vi "S&E Monitor.vi"(1 "Action(GET 250)":T3=enum."Get last  250", 5 "Type":T1, 7 "E&S Message in":T2, 11 "error in (no error)":errorcluster, 12 "Numb Alarm(250)":i32=250) -> (8 "S&E":T2[](array[typedef]), 15 "error out":errorcluster)   [LabVIEW 2011]
uses:
  Actino S&E monitor.ctl
  emi Lib/System 01/0 - General/S&E reporting/Private/_emi_ S&E Message.ctl
  emi Lib/System 01/0 - General/S&E reporting/Private/_emi_ S&E Message type.ctl
  reate/S&E Analog Alarm type.ctl
  GUI/Status Indikator Helper.ctl
  reate/S&E Digital Alarm Type.ctl
  Measurments Handling/Status Digitalish.ctl
  <vilib>/Utility/VariantDataType/GetNumericInfo.vi
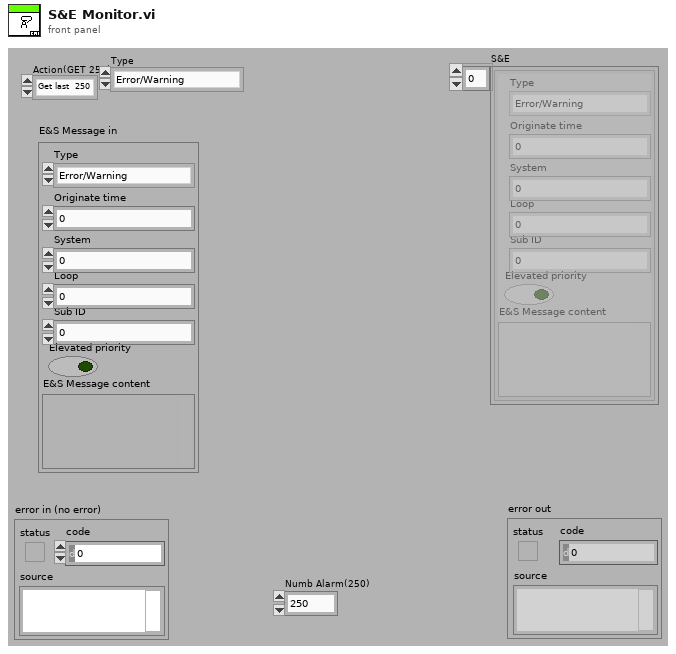
[diagram p1: front panel]
types:
  T1 = typedef "_emi_ S&E Message type.ctl" = enum16{"Error/Warning", "Note", "Debug", "Event", "Alarm Analog", "Alarm Digital", "Annotation"}
  T2 = typedef "_emi_ S&E Message.ctl" = cluster{"Type":T1, "Originate time":dbl, "System":u8, "Loop":u16, "Sub ID":u16, "Elevated priority":bool, "E&S Message content":variant}
  T3 = typedef "Actino S&E monitor.ctl" = enum16{"GET(type history)", "SET S&E", "(Re)Init", "Get Error state", "Get  Alarm state", "Get All", "Get last  250", "Get Alarm History"}
  T4 = typedef "S&E Analog Alarm type.ctl" = cluster{"Alarm":bool, "State":T5, "Value":dbl, "Source name":string}
  T5 = typedef "Status Indikator Helper.ctl" = enum16{"Norm", "L", "H", "LL", "HH", "Value", "Technical"}
  T6 = typedef "S&E Digital Alarm Type.ctl" = cluster{"Alarm":bool, "Enum":T5, "Value":T7, "Source name":string, "Status text":string}
  T7 = typedef "Status Digitalish.ctl" = enum16{"NA", "False", "True"}
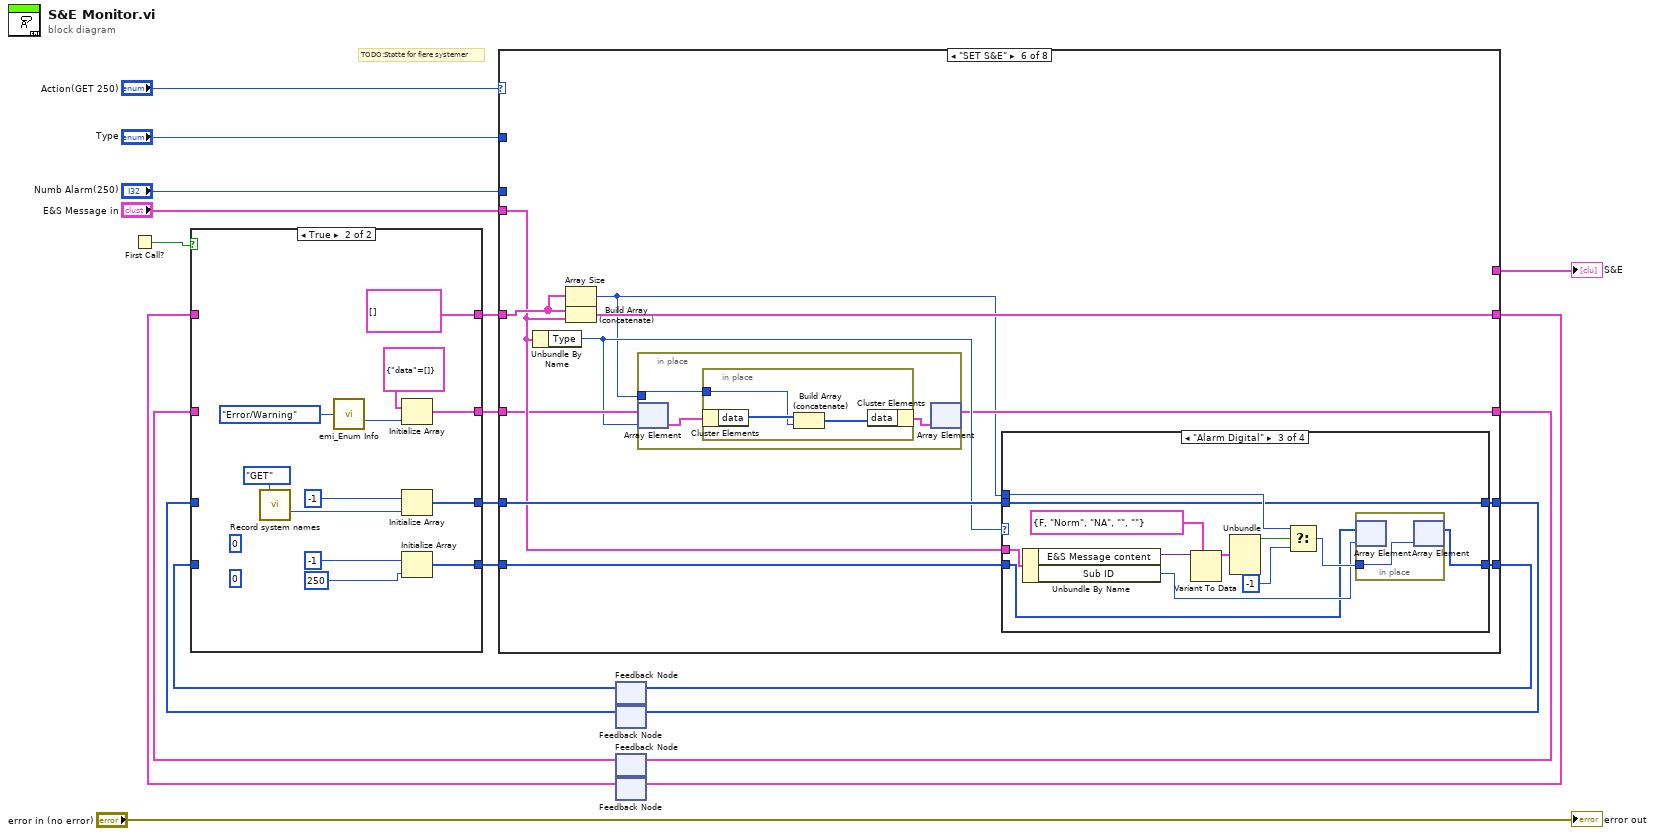
[diagram p0: block diagram]
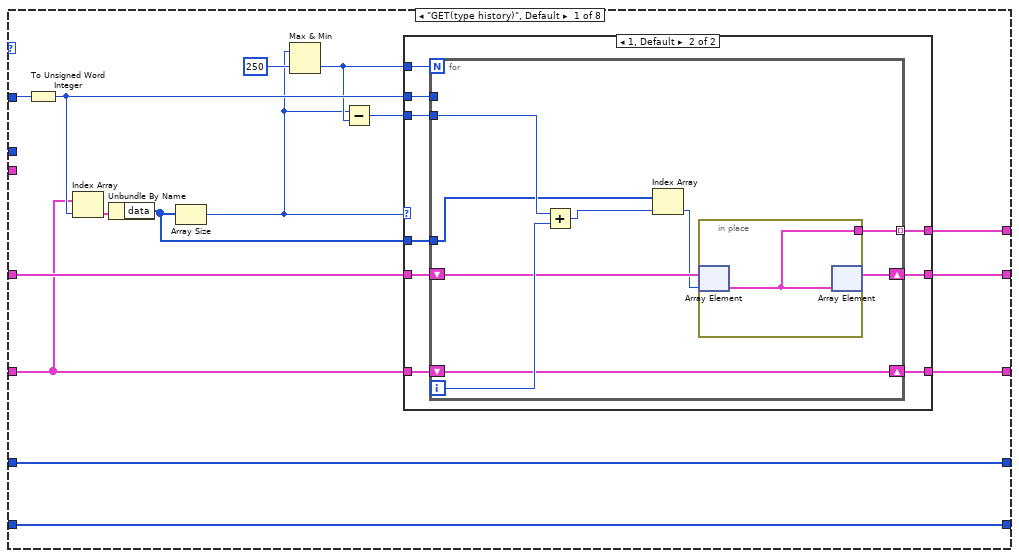
[diagram p3: hidden frame]
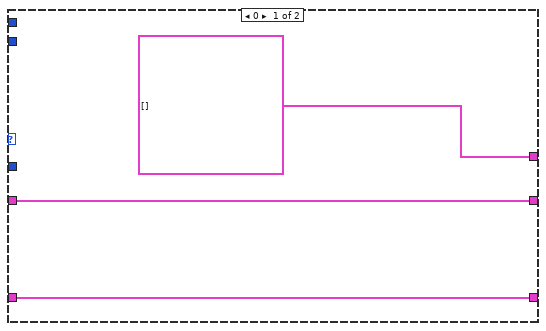
[diagram p4: hidden frame]
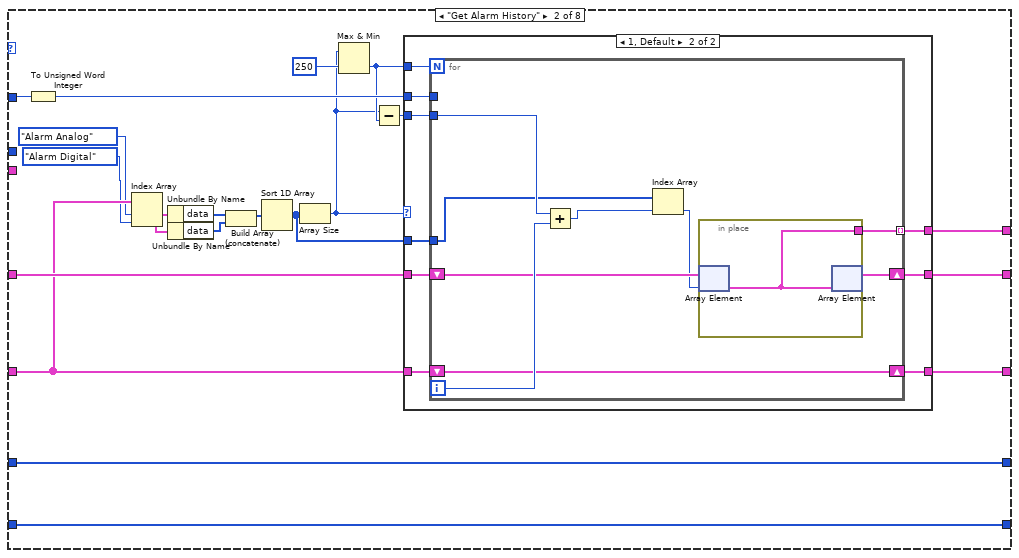
[diagram p5: hidden frame]
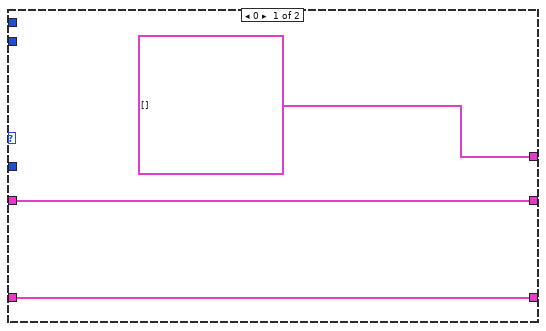
[diagram p6: hidden frame]
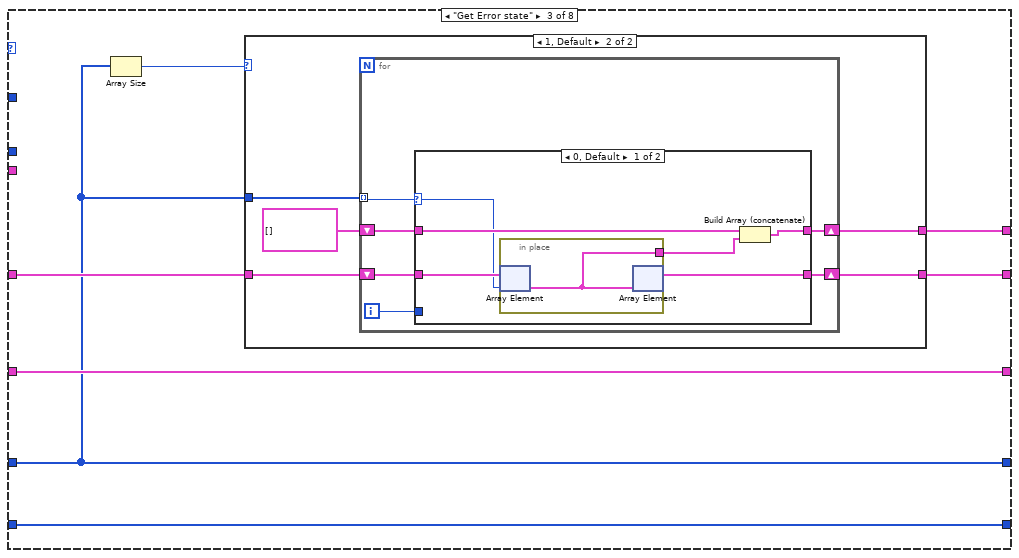
[diagram p7: hidden frame]
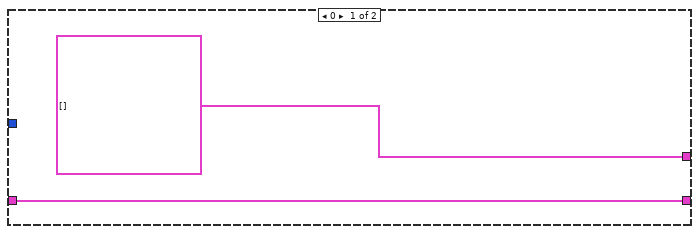
[diagram p8: hidden frame]
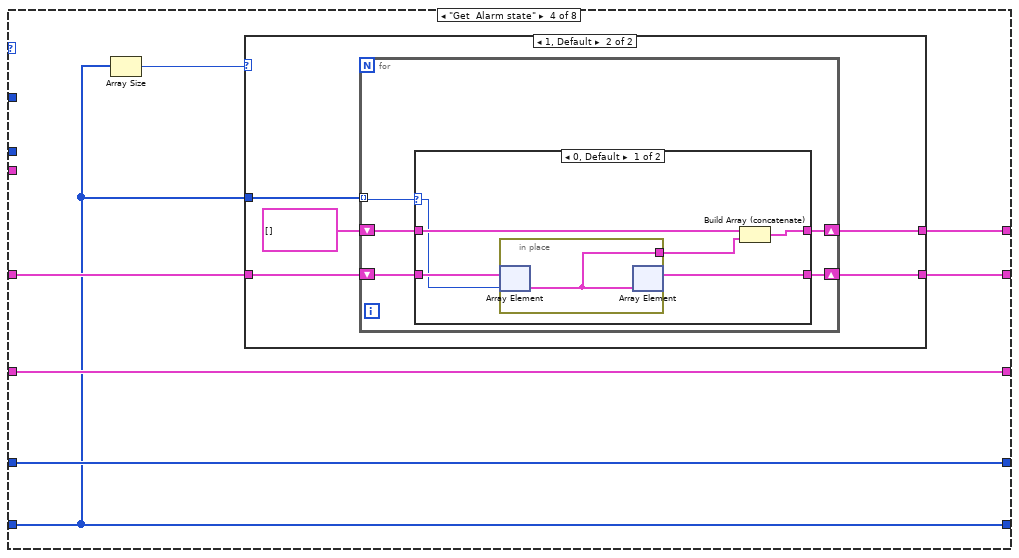
[diagram p10: hidden frame]
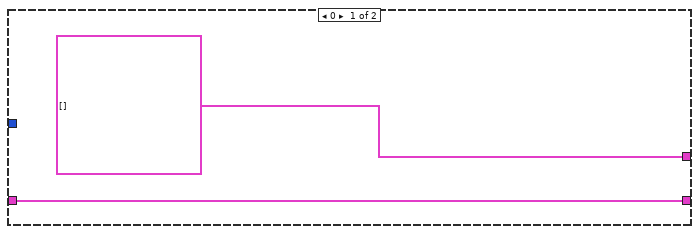
[diagram p11: hidden frame]
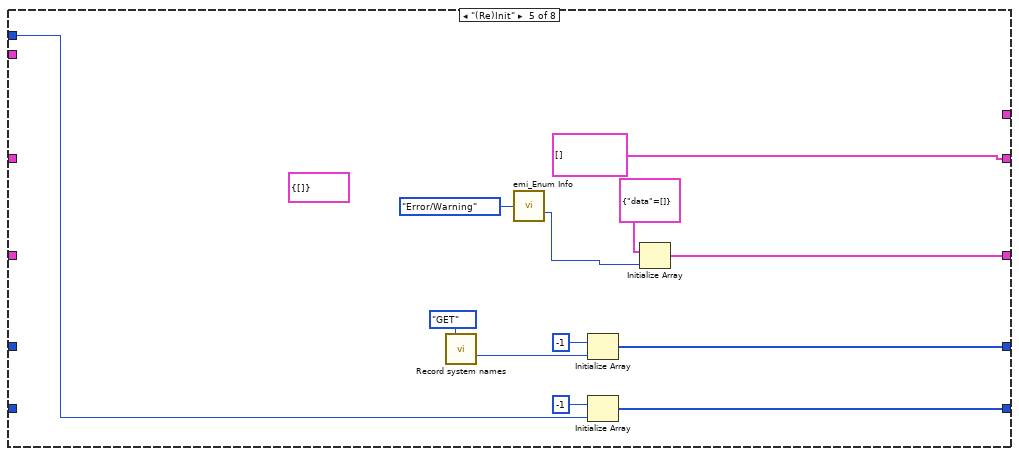
[diagram p13: hidden frame]
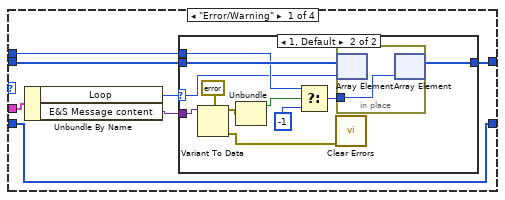
[diagram p14: hidden frame]
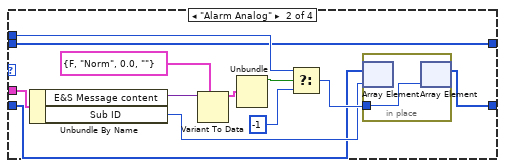
[diagram p16: hidden frame]
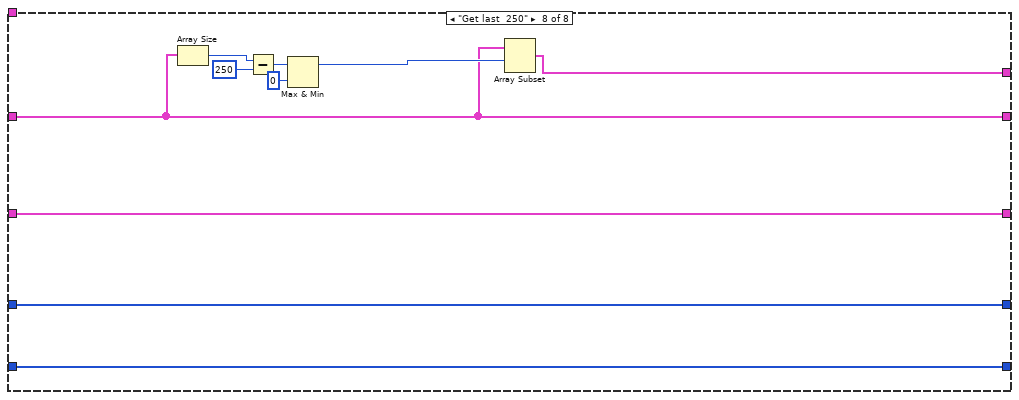
[diagram p19: hidden frame]
diagram:
  # "TODO:Støtte for flere systemer"
  n1 = First Call?() -> (First Call?: T/F=w16:bool)
  n2 = feedback #1() -> (w2:i32[])  [unwired: 1 in]
  n3 = feedback #2() -> (w6:i32[])  [unwired: 1 in]
  n4 = feedback #3() -> (w10:cluster{"data":i32[]}[])  [unwired: 1 in]
  n5 = feedback #4() -> (w17:T2[])  [unwired: 1 in]
  n6 = case shown="True" w16 {
    tunnel: w17 -> [w23 _]
    tunnel: [w23 T2[] []] -> w14
    tunnel: [w20 w33] -> w11
    tunnel: w10 -> [w20 _]
    tunnel: [w22 w28] -> w8
    tunnel: w6 -> [w22 _]
    tunnel: [w21 w27] -> w4
    tunnel: w2 -> [w21 _]
    frame False {
    }
    frame True {
      (unwired) 0 ("dimension size")
      (unwired) 0
      n7 = call "Record system names.vi"("Action(GET)"=enum16{"GET", "SET/Init"}."GET") -> ("Numb Loops in system"=w30:i32)  [unwired: 10 in, 4 out]
      n8 = call "emi_Enum Info.vi"("Enum"=_emi__S&E_Message_type."Error/Warning" ("Type")) -> ("Numb Elements"=w32:i32)  [unwired: 11 in, 3 out]
      n9 = Initialize Array(cluster{"data":i32[]} {"data"=[]}, w32) -> (w33:cluster{"data":i32[]}[])
      n10 = Initialize Array(-1, w30) -> (w28:i32[])
      n11 = Initialize Array(-1, 250 ("dimension size")) -> (w27:i32[])
    }
  }
  n12 = case shown="\"SET S&E\"" "Action(GET 250)" {
    tunnel: [w45 w88 w120 w150 T2[] [] w195 w250 w255] -> w15
    tunnel: w14 -> [w46 w89 w121 w151 _ w194 w250 w255]
    tunnel: "E&S Message in" -> [_ _ _ _ _ w191 _ _]
    tunnel: [w44 w87 w118 w148 w174 w186 w253 w263] -> w12
    tunnel: w11 -> [w39 w82 w118 w148 _ w188 w253 w263]
    tunnel: "Type" -> [w48 w91 _ _ _ _ _ _]
    tunnel: w8 -> [w50 w93 w116 w146 _ w192 w252 w262]
    tunnel: [w50 w93 w116 w146 w179 w193 w252 w262] -> w7
    tunnel: "Numb Alarm(250)" -> [_ _ _ _ w177 _ _ _]
    tunnel: w4 -> [w49 w92 w122 w145 _ w189 w251 w261]
    tunnel: [w49 w92 w122 w145 w176 w190 w251 w261] -> w3
    tunnel: [w42 w85 w119 w149 _ _ w250 w254] -> w1
    frame "GET(type history)", Default {
      n13 = To Unsigned Word Integer(number=w48) -> (unsigned 16bit integer=w43:u16)
      n14 = Index Array(array=w39, index=w43) -> (element=w38:cluster{"data":i32[]})
      n15 = Unbundle By Name(w38) -> ("data"=w36:i32[])
      n16 = Array Size(array=w36) -> (size(s)=w37:i32)
      n17 = Max & Min(x=w37, y=250) -> (min(x,y)=w41:i32)  [unwired: 1 out]
      n18 = Subtract(x=w37, y=w41) -> (x-y=w40:i32)
      n19 = case shown="1, Default" w37 {
        tunnel: w46 -> [w53 w62]
        tunnel: [w53 w61] -> w45
        tunnel: w39 -> [w52 w60]
        tunnel: [w52 w59] -> w44
        tunnel: w41 -> [_ w58]
        tunnel: w43 -> [_ w57]
        tunnel: [T2[] [] w56] -> w42
        tunnel: w40 -> [_ w55]
        tunnel: w36 -> [_ w54]
        frame 0 {
        }
        frame 1, Default {
          n20 = for {
            N: w58 -> [_]
            shift-right: [w70] -> w59
            shift-left: w60 -> [w70]
            shift-right: [w67] -> w61
            shift-left: w62 -> [w69]
            tunnel: w57 -> [_]
            tunnel: [w66] -> w56 mode=indexing
            tunnel: w55 -> [w65]
            tunnel: w54 -> [w64]
            i -> [w71]
            n21 = Add(x=w65, y=w71) -> (x+y=w63:i32)
            n22 = Index Array(array=w64, index=w63) -> (element=w68:i32)
            n23 = in-place {
              in-place-border: [w72] -> w66
              n24 = in-place-array #5(w69, w68) -> (w72:T2)
              n25 = in-place-array #5(w72) -> (w67:T2[])  [unwired: 1 out]
            }
          }
        }
      }
    }
    frame "Get Alarm History" {
      n26 = To Unsigned Word Integer(number=w91) -> (unsigned 16bit integer=w86:u16)
      n27 = Index Array(array=w82, index #1=_emi__S&E_Message_type."Alarm Analog" ("Type"), index #2=_emi__S&E_Message_type."Alarm Digital" ("Type")) -> (element #1=w81:cluster{"data":i32[]}, element #2=w77:cluster{"data":i32[]})
      n28 = Unbundle By Name(w81) -> ("data"=w76:i32[])
      n29 = Unbundle By Name(w77) -> ("data"=w75:i32[])
      n30 = Build Array (concatenate)(w76, w75) -> (w74:i32[])
      n31 = Sort 1D Array(array=w74) -> (sorted array=w73:i32[])
      n32 = Array Size(array=w73) -> (size(s)=w80:i32)
      n33 = Max & Min(x=w80, y=250) -> (min(x,y)=w84:i32)  [unwired: 1 out]
      n34 = Subtract(x=w80, y=w84) -> (x-y=w83:i32)
      n35 = case shown="1, Default" w80 {
        tunnel: w89 -> [w96 w105]
        tunnel: [w96 w104] -> w88
        tunnel: w82 -> [w95 w103]
        tunnel: [w95 w102] -> w87
        tunnel: w84 -> [_ w101]
        tunnel: w86 -> [_ w100]
        tunnel: [T2[] [] w99] -> w85
        tunnel: w83 -> [_ w98]
        tunnel: w73 -> [_ w97]
        frame 0 {
        }
        frame 1, Default {
          n36 = for {
            N: w101 -> [_]
            shift-right: [w113] -> w102
            shift-left: w103 -> [w113]
            shift-right: [w110] -> w104
            shift-left: w105 -> [w112]
            tunnel: w100 -> [_]
            tunnel: [w109] -> w99 mode=indexing
            tunnel: w98 -> [w108]
            tunnel: w97 -> [w107]
            i -> [w114]
            n37 = Add(x=w108, y=w114) -> (x+y=w106:i32)
            n38 = Index Array(array=w107, index=w106) -> (element=w111:i32)
            n39 = in-place {
              in-place-border: [w115] -> w109
              n40 = in-place-array #6(w112, w111) -> (w115:T2)
              n41 = in-place-array #6(w115) -> (w110:T2[])  [unwired: 1 out]
            }
          }
        }
      }
    }
    frame "Get Error state" {
      n42 = Array Size(array=w116) -> (size(s)=w117:i32)
      n43 = case shown="1, Default" w117 {
        tunnel: w121 -> [w124 w129]
        tunnel: [w124 w128] -> w120
        tunnel: [T2[] [] w127] -> w119
        tunnel: w116 -> [_ w126]
        frame 0 {
        }
        frame 1, Default {
          n44 = for {
            shift-right: [w134] -> w128
            shift-left: w129 -> [w135]
            tunnel: w126 -> [w132] mode=indexing
            shift-right: [w133] -> w127
            shift-left: T2[] [] -> [w131]
            i -> [w130]
            n45 = case shown="0, Default" w132 {
              selector: w132 -> [w136 _]
              tunnel: w135 -> [w141 w144]
              tunnel: [w140 w144] -> w134
              tunnel: [w138 w143] -> w133
              tunnel: w131 -> [w137 w143]
              tunnel: w130 -> [_ _]
              frame 0, Default {
                n46 = in-place {
                  in-place-border: [w142] -> w139
                  n47 = in-place-array #7(w141, w136) -> (w142:T2)
                  n48 = in-place-array #7(w142) -> (w140:T2[])  [unwired: 1 out]
                }
                n49 = Build Array (concatenate)(w137, w139) -> (w138:T2[])
              }
              frame -1 {
              }
            }
          }
        }
      }
    }
    frame "Get  Alarm state" {
      n50 = Array Size(array=w145) -> (size(s)=w147:i32)
      n51 = case shown="1, Default" w147 {
        tunnel: w151 -> [w153 w158]
        tunnel: [w153 w157] -> w150
        tunnel: [T2[] [] w156] -> w149
        tunnel: w145 -> [_ w155]
        frame 0 {
        }
        frame 1, Default {
          n52 = for {
            shift-right: [w162] -> w157
            shift-left: w158 -> [w163]
            tunnel: w155 -> [w160] mode=indexing
            shift-right: [w161] -> w156
            shift-left: T2[] [] -> [w159]
            n53 = case shown="0, Default" w160 {
              selector: w160 -> [w164 _]
              tunnel: w163 -> [w169 w172]
              tunnel: [w168 w172] -> w162
              tunnel: [w166 w171] -> w161
              tunnel: w159 -> [w165 w171]
              frame 0, Default {
                n54 = in-place {
                  in-place-border: [w170] -> w167
                  n55 = in-place-array #8(w169, w164) -> (w170:T2)
                  n56 = in-place-array #8(w170) -> (w168:T2[])  [unwired: 1 out]
                }
                n57 = Build Array (concatenate)(w165, w167) -> (w166:T2[])
              }
              frame -1 {
              }
            }
          }
        }
      }
    }
    frame "(Re)Init" {
      (unwired) cluster{i32[]} {[]}
      n58 = call "Record system names.vi"("Action(GET)"=enum16{"GET", "SET/Init"}."GET") -> ("Numb Loops in system"=w183:i32)  [unwired: 10 in, 4 out]
      n59 = call "emi_Enum Info.vi"("Enum"=_emi__S&E_Message_type."Error/Warning" ("Type")) -> ("Numb Elements"=w173:i32)  [unwired: 11 in, 3 out]
      n60 = Initialize Array(-1, w183) -> (w179:i32[])
      n61 = Initialize Array(-1, w177) -> (w176:i32[])
      n62 = Initialize Array(cluster{"data":i32[]} {"data"=[]}, w173) -> (w174:cluster{"data":i32[]}[])
    }
    frame "SET S&E" {
      n63 = Unbundle By Name(w191) -> ("Type"=w187:T1)
      n64 = Array Size(array=w194) -> (size(s)=w185:i32)
      n65 = Build Array (concatenate)(w194, w191) -> (w195:T2[])
      n66 = in-place {
        in-place-border: w185 -> [w197]
        n67 = in-place-array #9(w188, w187) -> (w198:cluster{"data":i32[]})
        n68 = in-place {
          in-place-border: w197 -> [w199]
          n69 = in-place-cluster #10(w198) -> ("data"=w201:i32[])
          n70 = Build Array (concatenate)(w201, w199) -> (w200:i32[])
          n71 = in-place-cluster #10("data"=w200) -> (w196:cluster{"data":i32[]})
        }
        n72 = in-place-array #9(w196) -> (w186:cluster{"data":i32[]}[])  [unwired: 1 out]
      }
      n73 = case shown="\"Alarm Digital\"" w187 {
        tunnel: [w206 w226 w239 w249] -> w193
        tunnel: w192 -> [w207 w226 w239 w249]
        tunnel: w185 -> [w204 w229 w242 _]
        tunnel: w191 -> [w208 w233 w246 _]
        tunnel: [w203 w223 w236 w248] -> w190
        tunnel: w189 -> [w203 w224 w237 w248]
        frame "Error/Warning" {
          n74 = Unbundle By Name(w208) -> ("Loop"=w202:u16, "E&S Message content"=w205:variant)
          n75 = case shown="1, Default" w202 {
            selector: w202 -> [_ w211]
            tunnel: w207 -> [w209 w220]
            tunnel: [w209 w219] -> w206
            tunnel: w205 -> [_ w218]
            tunnel: w204 -> [_ w214]
            frame 9999 {
            }
            frame 1, Default {
              n76 = Variant To Data(type=errorcluster {"status"=FALSE, "code"=0, "source"=""} ("error in (no error)"), Variant=w218) -> (data=w216:errorcluster, error out=w210:errorcluster)  [unwired: 1 in]
              n77 = Unbundle(w216) -> ("status"=w215:bool)  [unwired: 2 out]
              n78 = Select(t=w214, s=w215, f=-1) -> (s? t:f=w213:i32)
              n79 = call <vilib>:"Clear Errors.vi"("error in (no error)"=w210) -> ()  [unwired: 6 in, 1 out]
              n80 = in-place {
                in-place-border: w213 -> [w221]
                n81 = in-place-array #11(w220, w211) -> ()  [unwired: 1 out]
                n82 = in-place-array #11(w221) -> (w219:i32[])  [unwired: 1 out]
              }
            }
          }
        }
        frame "Alarm Analog" {
          n83 = Unbundle By Name(w233) -> ("E&S Message content"=w232:variant, "Sub ID"=w225:u16)
          n84 = Variant To Data(type=T4 {"Alarm"=FALSE, "State"=enum."Norm", "Value"=0.0, "Source name"=""} ("S&E Alarm"), Variant=w232) -> (data=w231:T4)  [unwired: 1 in, 1 out]
          n85 = Unbundle(w231) -> ("Alarm"=w230:bool)  [unwired: 3 out]
          n86 = Select(t=w229, s=w230, f=-1) -> (s? t:f=w228:i32)
          n87 = in-place {
            in-place-border: w228 -> [w234]
            n88 = in-place-array #12(w224, w225) -> ()  [unwired: 1 out]
            n89 = in-place-array #12(w234) -> (w223:i32[])  [unwired: 1 out]
          }
        }
        frame "Alarm Digital" {
          n90 = Unbundle By Name(w246) -> ("E&S Message content"=w245:variant, "Sub ID"=w238:u16)
          n91 = Variant To Data(type=T6 {"Alarm"=FALSE, "Enum"=enum."Norm", "Value"=enum."NA", "Source name"="", "Status text"=""} ("S&E Alarm"), Variant=w245) -> (data=w244:T6)  [unwired: 1 in, 1 out]
          n92 = Unbundle(w244) -> ("Alarm"=w243:bool)  [unwired: 4 out]
          n93 = Select(t=w242, s=w243, f=-1) -> (s? t:f=w241:i32)
          n94 = in-place {
            in-place-border: w241 -> [w247]
            n95 = in-place-array #13(w237, w238) -> ()  [unwired: 1 out]
            n96 = in-place-array #13(w247) -> (w236:i32[])  [unwired: 1 out]
          }
        }
        frame "Note", Default {
        }
      }
    }
    frame "Get All" {
    }
    frame "Get last  250" {
      n97 = Array Size(array=w255) -> (size(s)=w260:i32)
      n98 = Subtract(x=w260, y=250) -> (x-y=w258:i32)
      n99 = Max & Min(x=w258, y=0) -> (max(x,y)=w256:i32)  [unwired: 1 out]
      n100 = Array Subset(array=w255, index=w256) -> (w254:T2[])  [unwired: 1 in]
    }
  }
  "S&E" <- w1
  n101 = feedback-in #1(w3) -> ()
  n102 = feedback-in #2(w7) -> ()
  n103 = feedback-in #3(w12) -> ()
  n104 = feedback-in #4(w15) -> ()
  "error out" <- "error in (no error)"
